vi "CRYFlatten Work State.vi"() -> (3 "work state # flattened":string)   [LabVIEW 2013]
uses:
  CRYSystem/Hardware/CRYHardware Global.vi
  CRYSystem/Calibration/SubVI/CRYCal Global.vi
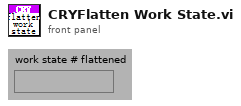
[diagram p1: front panel]
types:
  T1 = cluster{"Mic Vol-L":dbl, "Mic Vol-R":dbl, "Mic Res-L":dbl, "Mic Res-R":dbl, "Cal. Input other":dbl, "Ref. Freq. other":dbl}
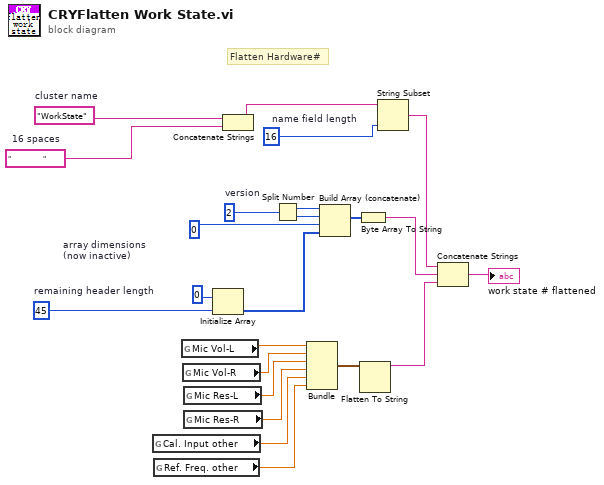
[diagram p0: block diagram]
diagram:
  w22 = u8 0  # array dimensions (now inactive)
  w19 = 16  # name field length
  w18 = "                "  # 16 spaces
  w17 = "WorkState"  # cluster name
  w12 = 45  # remaining header length
  w8 = u16 2  # version
  # "Flatten Hardware#"
  n1 = global read "CRYCal Global.vi" "Cal. Input other"() -> (w2:dbl)
  n2 = global read "CRYCal Global.vi" "Ref. Freq. other"() -> (w1:dbl)
  n3 = global read "CRYHardware Global.vi" "Mic Vol-L"() -> (w7:dbl)
  n4 = global read "CRYHardware Global.vi" "Mic Vol-R"() -> (w6:dbl)
  n5 = global read "CRYHardware Global.vi" "Mic Res-L"() -> (w5:dbl)
  n6 = global read "CRYHardware Global.vi" "Mic Res-R"() -> (w4:dbl)
  n7 = Initialize Array(u8 0, w12) -> (w16:u8[])
  n8 = Concatenate Strings(w17, w18) -> (w20:string)
  n9 = Split Number(x=w8) -> (hi(x)=w9:u8, lo(x)=w10:u8)
  n10 = Bundle("Mic Vol-L"=w7, "Mic Vol-R"=w6, "Mic Res-L"=w5, "Mic Res-R"=w4, "Cal. Input other"=w2, "Ref. Freq. other"=w1) -> (w3:T1)  [unwired: 1 in]
  n11 = Build Array (concatenate)(w9, w10, w22, w16) -> (w13:u8[])
  n12 = Byte Array To String(unsigned byte array=w13) -> (string=w15:string)
  n13 = Flatten To String(anything=w3) -> (data string=w23:string)  [unwired: 1 in, 4 out]
  n14 = String Subset(string=w20, length (rest)=w19) -> (substring=w21:string)  [unwired: 1 out]
  n15 = Concatenate Strings(w21, w15, w23) -> (→"work state # flattened":string)
